vi "Get Visa References by Model.vi"(8 "error in":errorcluster, 10 "Search Mode":T1 items=["Canonical Names Only"=0, "Aliases Only"=2, "Include Matching Aliases"=3, "Include All Aliases"=4], 11 "Model":string) -> (0 "error out":errorcluster, 3 "Model References":refnum<visa-resource-name>[](array[refnum]))   [LabVIEW 2021, in "Keysight U1282A.lvlib"]
doc: "Simple string based state machine.\n\n--------------------\n<Author>\n<Company>"
uses:
  Keysight U1282A.lvlib
  <vilib>/Instr/_visa.llb/VISA Find Search Mode.ctl
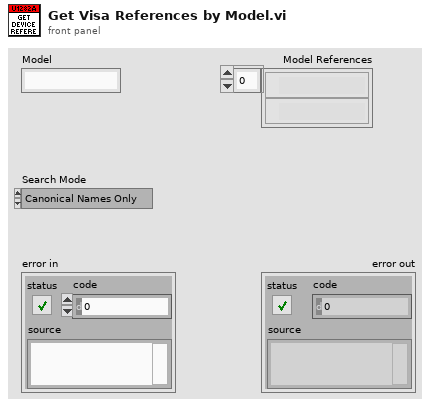
[diagram p1: front panel]
types:
  T1 = typedef "VISA Find Search Mode.ctl" = u32
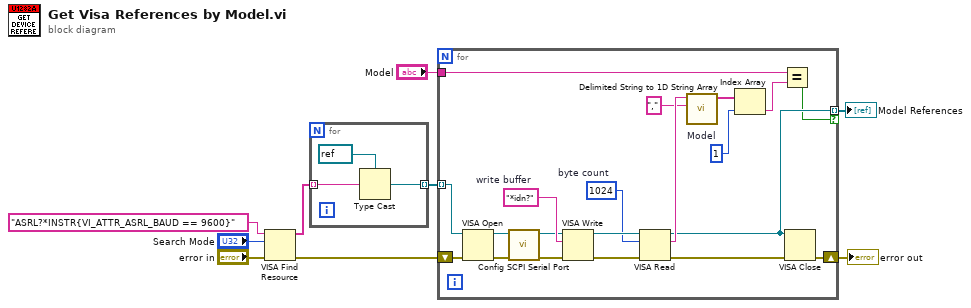
[diagram p0: block diagram]
diagram:
  n1 = VISA Find Resource(8:"error in", 10:"Search Mode", 11:"ASRL?*INSTR{VI_ATTR_ASRL_BAUD == 9600}" ("expression (\"?*\")")) -> (0:w2:errorcluster, 3:w7:string[])  [unwired: 1 out]
  n2 = for {
    tunnel: w7 -> [w12] mode=indexing
    tunnel: [w10] -> w8 mode=indexing
    n3 = Type Cast(type=refnum<visa-resource-name> refnum ("VISA resource name"), x=w12) -> (*(type *) &x=w10:refnum<visa-resource-name>)
  }
  n4 = for {
    tunnel: w8 -> [w21] mode=indexing
    shift-right: [w31] -> w4
    shift-left: w2 -> [w32]
    tunnel: [w14] -> w5 mode=indexing if=w13
    tunnel: "Model" -> [w15]
    w19 = 1  # Model
    w26 = u32 1024  # byte count
    w27 = "*idn?"  # write buffer
    n5 = VISA Open(error in (no error)=w32, VISA resource name=w21) -> (VISA resource name=w22:refnum<visa-resource-name>, error out=w23:errorcluster)  [unwired: 3 in]
    n6 = call "Config SCPI Serial Port.vi"("error in"=w23, "VISA Refnum in"=w22) -> ("error out"=w24:errorcluster, "VISA Refnum out"=w25:refnum<visa-resource-name>)  [unwired: 8 in]
    n7 = VISA Write(VISA resource name=w25, write buffer=w27, error in (no error)=w24) -> (VISA resource name out=w28:refnum<visa-resource-name>, error out=w30:errorcluster)  [unwired: 1 out]
    n8 = VISA Read(VISA resource name=w28, byte count=w26, error in (no error)=w30) -> (VISA resource name out=w14:refnum<visa-resource-name>, read buffer=w20:string, error out=w29:errorcluster)  [unwired: 1 out]
    n9 = call <vilib>:"Delimited String to 1D String Array.vi"("delimiter"=",", "delimited string"=w20) -> ("string array"=w18:string[])  [unwired: 9 in]
    n10 = Index Array(array=w18, index=w19) -> (element=w16:string)
    n11 = Equal?(x=w15, y=w16) -> (x = y?=w13:bool)
    n12 = VISA Close(VISA resource name=w14, error in (no error)=w29) -> (error out=w31:errorcluster)
  }
  "Model References" <- w5
  "error out" <- w4
